vi "Read Circle.vi"   [LabVIEW 2011, in "LMH-Leap.lvlib"]
doc: "Read all data from circle gestures. Use the polymorphic instance to select between one or N circle gestures."
uses:
  LMH-Leap.lvlib
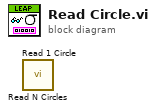
[diagram p0: block diagram]
diagram:
  n1 = call "Read N Circles.vi"() -> ()  [unwired: 8 in, 4 out]
  n2 = call "Read 1 Circle.vi"() -> ()  [unwired: 8 in, 4 out]
